vi "串口.vi"(9 "字符串":string, 10 "VISA resource name":refnum<visa-resource-name> caption="VISA资源名称") -> ()   [LabVIEW 2018]
uses:
  <vilib>/Instr/_visa.llb/VISA Configure Serial Port (Instr).vi
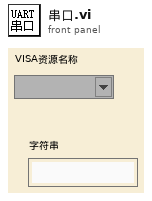
[diagram p1: front panel]
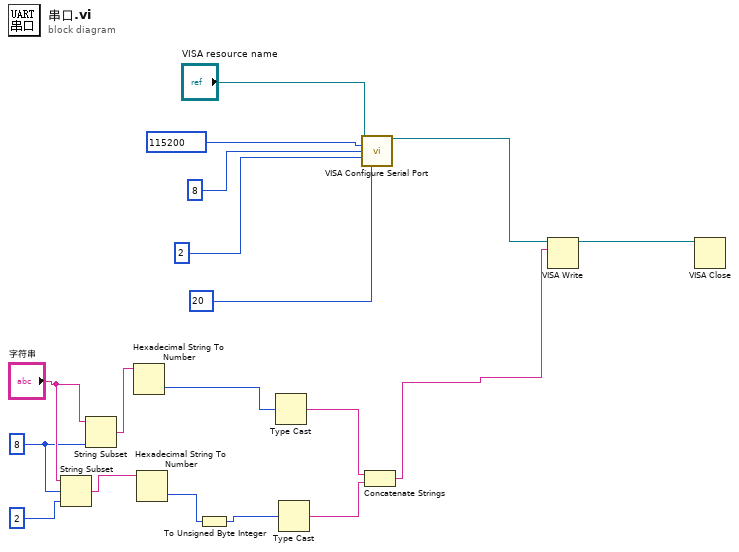
[diagram p0: block diagram]
diagram:
  w3 = 8
  n1 = String Subset(string="字符串", offset (0)=w3, length (rest)=2) -> (substring=w5:string)
  n2 = String Subset(string="字符串", length (rest)=w3) -> (substring=w6:string)  [unwired: 1 in]
  n3 = Hexadecimal String To Number(string=w6) -> (number=w11:u32)  [unwired: 2 in, 1 out]
  n4 = Hexadecimal String To Number(string=w5) -> (number=w2:u32)  [unwired: 2 in, 1 out]
  n5 = To Unsigned Byte Integer(number=w2) -> (unsigned 8bit integer=w1:u8)
  n6 = Type Cast(x=w11) -> (*(type *) &x=w10:string)  [unwired: 1 in]
  n7 = Type Cast(x=w1) -> (*(type *) &x=w9:string)  [unwired: 1 in]
  n8 = call-poly "VISA Configure Serial Port"("VISA resource name"="VISA resource name", "baud rate (9600)"=115200, "data bits (8)"=8, "parity (0:none)"=2, "stop bits (10: 1 bit)"=20) -> ("VISA resource name out"=w13:refnum<visa-resource-name>)  [unwired: 9 in, 1 out]
  n9 = Concatenate Strings(w10, w9) -> (w8:string)
  n10 = VISA Write(VISA resource name=w13, write buffer=w8) -> (VISA resource name out=w12:refnum<visa-resource-name>)  [unwired: 1 in, 2 out]
  n11 = VISA Close(VISA resource name=w12) -> ()  [unwired: 1 in, 1 out]
